vi "BaseProvider_WireStylesManager.vi"(7 "Action(Read)":enum16{"Read", "UpdateOne", "DeleteOne"}(ring), 8 "error in (no error)":errorcluster, 9 "NewIndex(-1=NoChange/Inserted Last If not found)":i32=-1, 10 "WireConfiguration(New or Updating)":T1={"Edge thickness"=1, "Edge color"=5667411, "Center thickness"=1, "Center pattern"=enum."Solid", "CenterColor1"=9740924, "CenterColor2"=8694662, "Tunnels and terminals colors"=131187}, 11 "WireStyleName(Default)":string="Default") -> (0 "error out":errorcluster, 1 "AllWireConfigurations":T1[](array[typedef]), 2 "AllWireConfigurations(Names)":string[](array[string]), 3 "SelectedWireConfiguration":T1={"Edge thickness"=1, "Edge color"=5667411, "Center thickness"=1, "Center pattern"=enum."Solid", "CenterColor1"=9740924, "CenterColor2"=8694662, "Tunnels and terminals colors"=131187})   [LabVIEW 2020]
uses:
  SubVIs/GOOP_WireConfigurationType.ctl
  SubVIs/GOOP_WirePattern.ctl
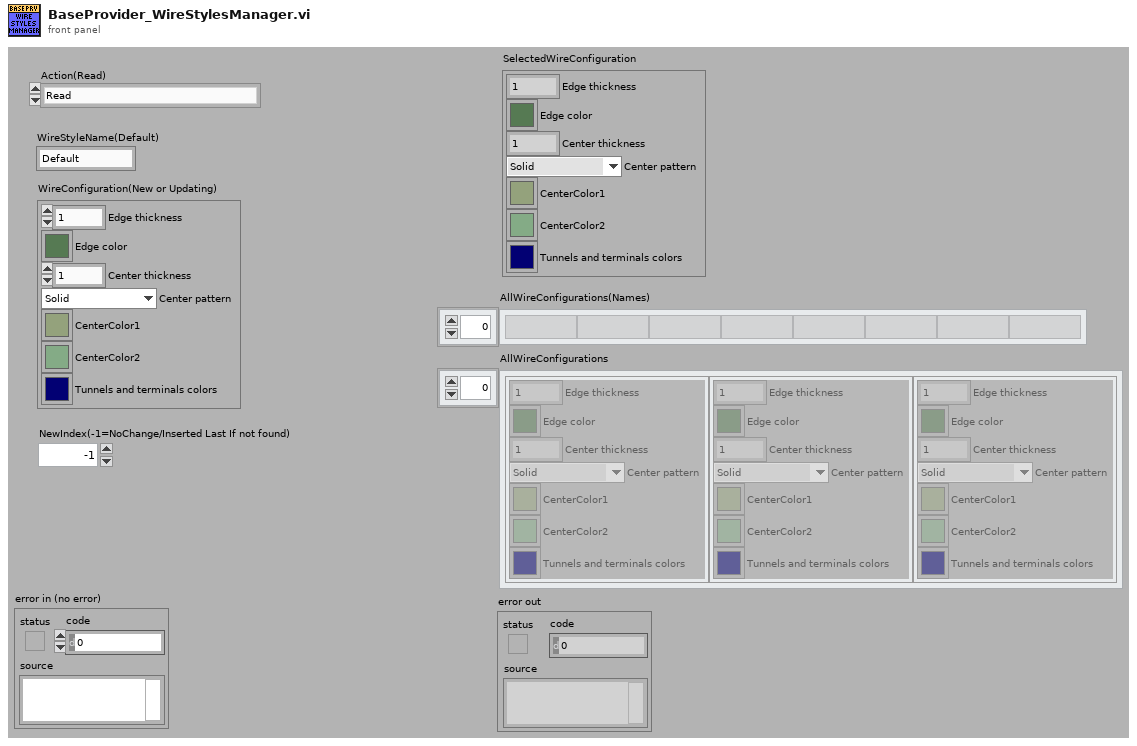
[diagram p1: front panel]
types:
  T1 = typedef "GOOP_WireConfigurationType.ctl" = cluster{"Edge thickness":i32, "Edge color":u32, "Center thickness":i32, "Center pattern":T2, "CenterColor1":u32, "CenterColor2":u32, "Tunnels and terminals colors":u32}
  T2 = typedef "GOOP_WirePattern.ctl" = enum16{"Solid", "Large dash", "Small dash"}
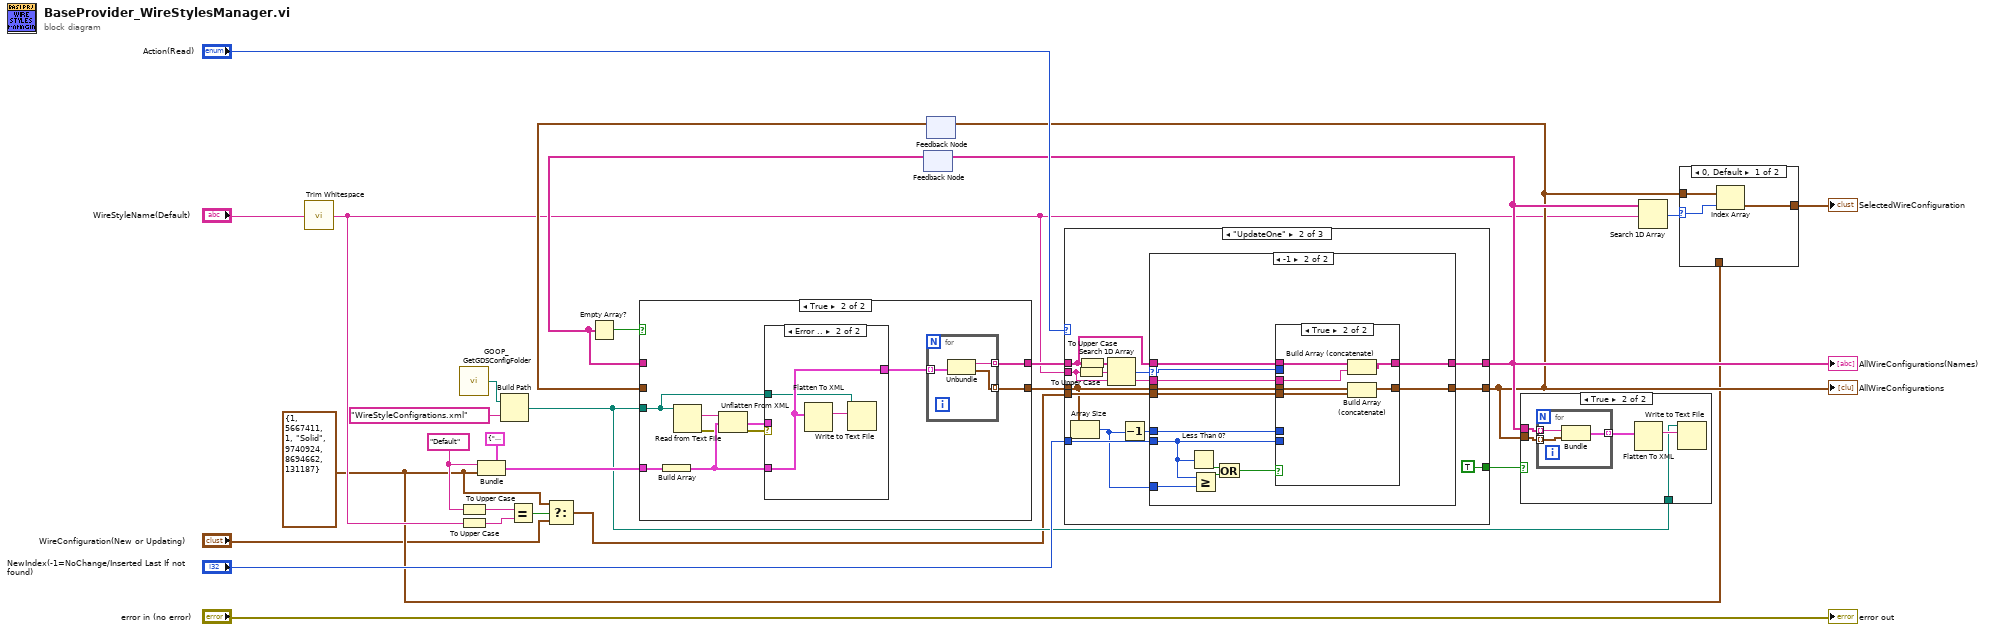
[diagram p0: block diagram]
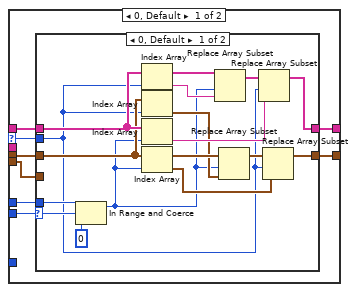
[diagram p4: hidden frame]
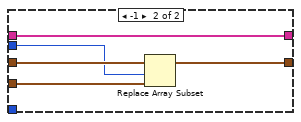
[diagram p5: hidden frame]
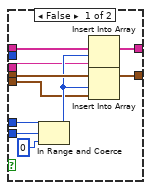
[diagram p6: hidden frame]
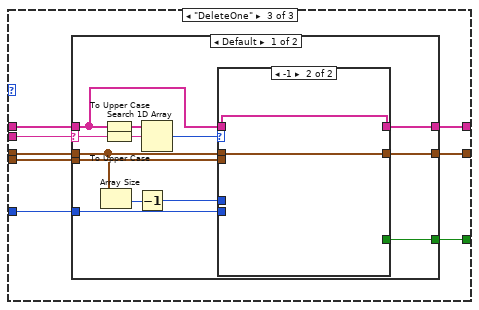
[diagram p7: hidden frame]
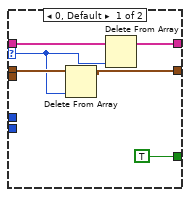
[diagram p8: hidden frame]
diagram:
  w8 = "Default" ("String")
  w3 = T1 {"Edge thickness"=1, "Edge color"=5667411, "Center thickness"=1, "Center pattern"=enum."Solid", "CenterColor1"=9740924, "CenterColor2"=8694662, "Tunnels and terminals colors"=131187} ("WireConfiguration")
  n1 = call <vilib>:"Trim Whitespace.vi"("string"="WireStyleName(Default)") -> ("trimmed string"=w7:string)  [unwired: 1 in]
  n2 = call "GOOP_GetGDSConfigFolder.vi"() -> ("GDSFolderPath"=w26:path)
  n3 = To Upper Case(1:w8) -> (0:w6:string)
  n4 = To Upper Case(1:w7) -> (0:w5:string)
  n5 = Bundle(cluster=cluster{"Name":string, "WireStyle":T1} {"Name"="", "WireStyle"={"Edge thickness"=0, "Edge color"=0, "Center thickness"=0, "Center pattern"=enum."Solid", "CenterColor1"=0, "CenterColor2"=0, "Tunnels and terminals colors"=0}} ("output cluster"), "Name"=w8, "WireStyle"=w3) -> (w23:cluster{"Name":string, "WireStyle":T1})
  n6 = Build Path(base path=w26, name or relative path="WireStyleConfigrations.xml") -> (appended path=w10:path)
  n7 = Equal?(x=w6, y=w5) -> (x = y?=w4:bool)
  n8 = Select(t=w3, s=w4, f="WireConfiguration(New or Updating)") -> (s? t:f=w1:T1)
  n9 = feedback #1() -> (w21:string[])  [unwired: 1 in]
  n10 = Empty Array?(array=w21) -> (empty?=w24:bool)
  n11 = feedback #2() -> (w22:T1[])  [unwired: 1 in]
  n12 = case shown="True" w24 {
    tunnel: w23 -> [_ w39]
    tunnel: w10 -> [_ w35]
    tunnel: [w29 w37] -> w17
    tunnel: [w28 w36] -> w16
    tunnel: w22 -> [w28 _]
    tunnel: w21 -> [w29 _]
    frame False {
    }
    frame True {
      n13 = Build Array(w39) -> (w38:cluster{"Name":string, "WireStyle":T1}[])
      n14 = Read from Text File(file (use dialog)=w35) -> (text=w32:string, error out=w34:errorcluster)  [unwired: 3 in, 2 out]
      n15 = Unflatten From XML(xml string=w32, type=w38, error in (no error)=w34) -> (value=w31:cluster{"Name":string, "WireStyle":T1}[], error out=w33:errorcluster)
      n16 = case shown="Error .." w33 {
        tunnel: [w43 w46] -> w30
        tunnel: w38 -> [_ w46]
        tunnel: w35 -> [_ w44]
        tunnel: w31 -> [w43 _]
        frame No Error {
        }
        frame Error {
          n17 = Flatten To XML(6:w46) -> (2:w45:string)
          n18 = Write to Text File(file (use dialog)=w44, text=w45) -> ()  [unwired: 2 in, 3 out]
        }
      }
      n19 = for {
        tunnel: w30 -> [w42] mode=indexing
        tunnel: [w41] -> w37 mode=indexing
        tunnel: [w40] -> w36 mode=indexing
        n20 = Unbundle(w42) -> ("Name"=w41:string, "WireStyle"=w40:T1)
      }
    }
  }
  n21 = case shown="\"UpdateOne\"" "Action(Read)" {
    tunnel: w17 -> [w48 w52 w124]
    tunnel: w16 -> [w47 w55 w120]
    tunnel: [w48 w58 w123] -> w12
    tunnel: [w47 w59 w125] -> w11
    tunnel: w7 -> [_ w56 w121]
    tunnel: "NewIndex(-1=NoChange/Inserted Last If not found)" -> [_ w60 w126]
    tunnel: w1 -> [_ w57 w122]
    tunnel: [_ TRUE w119] -> w9
    frame "Read", Default {
    }
    frame "UpdateOne" {
      n22 = Array Size(array=w55) -> (size(s)=w49:i32)
      n23 = To Upper Case(1:w56) -> (0:w51:string)
      n24 = To Upper Case(1:w52) -> (0:w50:string[])
      n25 = Search 1D Array(1D array=w50, element=w51) -> (index of element=w61:i32)  [unwired: 1 in]
      n26 = Decrement(x=w49) -> (x-1=w54:i32)
      n27 = case shown="-1" w61 {
        selector: w61 -> [w68 w96]
        tunnel: w60 -> [w65 w94]
        tunnel: w55 -> [w69 w102]
        tunnel: [w67 w100] -> w59
        tunnel: w52 -> [w64 w99]
        tunnel: [w63 w98] -> w58
        tunnel: w57 -> [w66 w101]
        tunnel: w56 -> [_ w97]
        tunnel: w54 -> [w62 w95]
        tunnel: w49 -> [_ w93]
        frame 0, Default {
          n28 = case shown="0, Default" w65 {
            selector: w65 -> [w83 _]
            tunnel: w69 -> [w78 w89]
            tunnel: w68 -> [w70 w88]
            tunnel: [w76 w87] -> w67
            tunnel: w66 -> [_ w86]
            tunnel: w64 -> [w81 w85]
            tunnel: [w79 w85] -> w63
            tunnel: w62 -> [w82 _]
            frame 0, Default {
              n29 = In Range and Coerce(upper limit=w82, x=w83, lower limit=0) -> (coerced(x)=w71:i32)  [unwired: 1 out]
              n30 = Index Array(array=w81, index=w70) -> (element=w75:string)
              n31 = Index Array(array=w78, index=w70) -> (element=w73:T1)
              n32 = Index Array(array=w81, index=w71) -> (element=w74:string)
              n33 = Index Array(array=w78, index=w71) -> (element=w72:T1)
              n34 = Replace Array Subset(array=w81, new element=w75, index=w71) -> (w80:string[])
              n35 = Replace Array Subset(array=w78, new element=w73, index=w71) -> (w77:T1[])
              n36 = Replace Array Subset(array=w80, new element=w74, index=w70) -> (w79:string[])
              n37 = Replace Array Subset(array=w77, new element=w72, index=w70) -> (w76:T1[])
            }
            frame -1 {
              n38 = Replace Array Subset(array=w89, new element=w86, index=w88) -> (w87:T1[])
            }
          }
        }
        frame -1 {
          n39 = Less Than 0?(x=w94) -> (x < 0?=w92:bool)
          n40 = Greater Or Equal?(x=w94, y=w93) -> (x >= y?=w91:bool)
          n41 = Or(x=w92, y=w91) -> (x .or. y?=w90:bool)
          n42 = case shown="True" w90 {
            tunnel: w102 -> [w109 w118]
            tunnel: w101 -> [w104 w117]
            tunnel: [w110 w116] -> w100
            tunnel: w99 -> [w112 w115]
            tunnel: [w111 w114] -> w98
            tunnel: w97 -> [w103 w113]
            tunnel: w96 -> [_ _]
            tunnel: w95 -> [w106 _]
            tunnel: w94 -> [w108 _]
            frame False {
              n43 = In Range and Coerce(upper limit=w106, x=w108, lower limit=0) -> (coerced(x)=w105:i32)  [unwired: 1 out]
              n44 = Insert Into Array(array=w112, index=w105, new element=w103) -> (w111:string[])
              n45 = Insert Into Array(array=w109, index=w105, new element=w104) -> (w110:T1[])
            }
            frame True {
              n46 = Build Array (concatenate)(w115, w113) -> (w114:string[])
              n47 = Build Array (concatenate)(w118, w117) -> (w116:T1[])
            }
          }
        }
      }
    }
    frame "DeleteOne" {
      n48 = case shown="Default" w121 {
        selector: w121 -> [w134 _]
        tunnel: w126 -> [w138 _]
        tunnel: [w137 w148] -> w125
        tunnel: w124 -> [w129 w149]
        tunnel: [w136 w149] -> w123
        tunnel: w122 -> [w135 _]
        tunnel: w120 -> [w133 w148]
        tunnel: [w130 _] -> w119
        frame Default {
          n49 = Array Size(array=w133) -> (size(s)=w132:i32)
          n50 = To Upper Case(1:w129) -> (0:w128:string[])
          n51 = To Upper Case(1:w134) -> (0:w127:string)
          n52 = Decrement(x=w132) -> (x-1=w131:i32)
          n53 = Search 1D Array(1D array=w128, element=w127) -> (index of element=w139:i32)  [unwired: 1 in]
          n54 = case shown="-1" w139 {
            selector: w139 -> [w141 _]
            tunnel: w138 -> [_ _]
            tunnel: w133 -> [w143 w146]
            tunnel: [w142 w146] -> w137
            tunnel: w129 -> [w145 w147]
            tunnel: [w144 w147] -> w136
            tunnel: w135 -> [_ _]
            tunnel: w131 -> [_ _]
            tunnel: [TRUE _] -> w130
            frame 0, Default {
              n55 = Delete From Array(array=w143, index=w141) -> (array with subset deleted=w142:T1[])  [unwired: 1 in, 1 out]
              n56 = Delete From Array(array=w145, index=w141) -> (array with subset deleted=w144:string[])  [unwired: 1 in, 1 out]
            }
            frame -1 {
            }
          }
        }
        frame "Default" {
        }
      }
    }
  }
  "AllWireConfigurations" <- w11
  "AllWireConfigurations(Names)" <- w12
  n57 = feedback-in #1(w12) -> ()
  n58 = feedback-in #2(w11) -> ()
  n59 = case shown="True" w9 {
    tunnel: w12 -> [_ w154]
    tunnel: w11 -> [_ w153]
    tunnel: w10 -> [_ w150]
    frame False {
    }
    frame True {
      n60 = for {
        tunnel: w154 -> [w157] mode=indexing
        tunnel: w153 -> [w156] mode=indexing
        tunnel: [w155] -> w151 mode=indexing
        n61 = Bundle("Name"=w157, "WireStyle"=w156) -> (w155:cluster{"Name":string, "WireStyle":T1})  [unwired: 1 in]
      }
      n62 = Flatten To XML(6:w151) -> (2:w152:string)
      n63 = Write to Text File(file (use dialog)=w150, text=w152) -> ()  [unwired: 2 in, 3 out]
    }
  }
  n64 = Search 1D Array(1D array=w12, element=w7) -> (index of element=w19:i32)  [unwired: 1 in]
  n65 = case shown="0, Default" w19 {
    selector: w19 -> [w159 _]
    tunnel: [w158 w161] -> w18
    tunnel: w3 -> [_ w161]
    tunnel: w11 -> [w160 _]
    frame 0, Default {
      n66 = Index Array(array=w160, index=w159) -> (element=w158:T1)
    }
    frame -1 {
    }
  }
  "SelectedWireConfiguration" <- w18
  "error out" <- "error in (no error)"
